vi "Update Non-SD Subpanel.vi"(7 "SubPanel Command":refnum<user-event>, 8 "error in (no error)":errorcluster, 9 "SubPanel Ref":refnum<vi>, 10 "SD Module in":refnum<class "SD Module.lvclass">, 11 "Node Ptr In":T1 format="%.0x") -> (0 "error out":errorcluster, 2 "SD Module out":refnum<class "SD Module.lvclass">, 3 "Node Ptr Out":T1 format="%.0x")   [LabVIEW 2017, in "Modules.lvlib" / "SD Module.lvclass"]
uses:
  SD Module.lvclass
  <vilib>/NI Veristand/Custom Device API/Custom Device Item Ref.ctl
  RSI Module/SubPanel Command.ctl
  <vilib>/Utility/miscctls.llb/LVRectTypeDef.ctl
  <vilib>/NI Veristand/Custom Device API/Custom Device API.lvlib
  RSI Module/RSI Module.lvclass
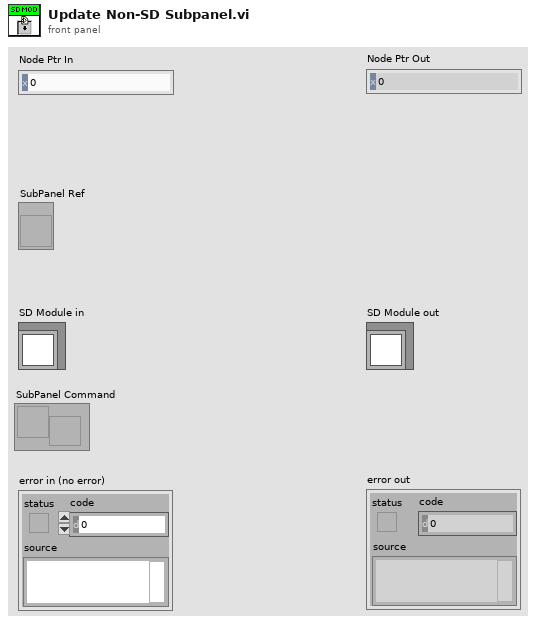
[diagram p1: front panel]
types:
  T1 = typedef "Custom Device API.lvlib/Custom Device Item Ref.ctl" = u64
  T2 = typedef "LVRectTypeDef.ctl" = cluster{"Left":i16, "Top":i16, "Right":i16, "Bottom":i16}
  T3 = typedef "LVBoundsTypeDef.ctl" = cluster{"Width":u32, "Height":u32}
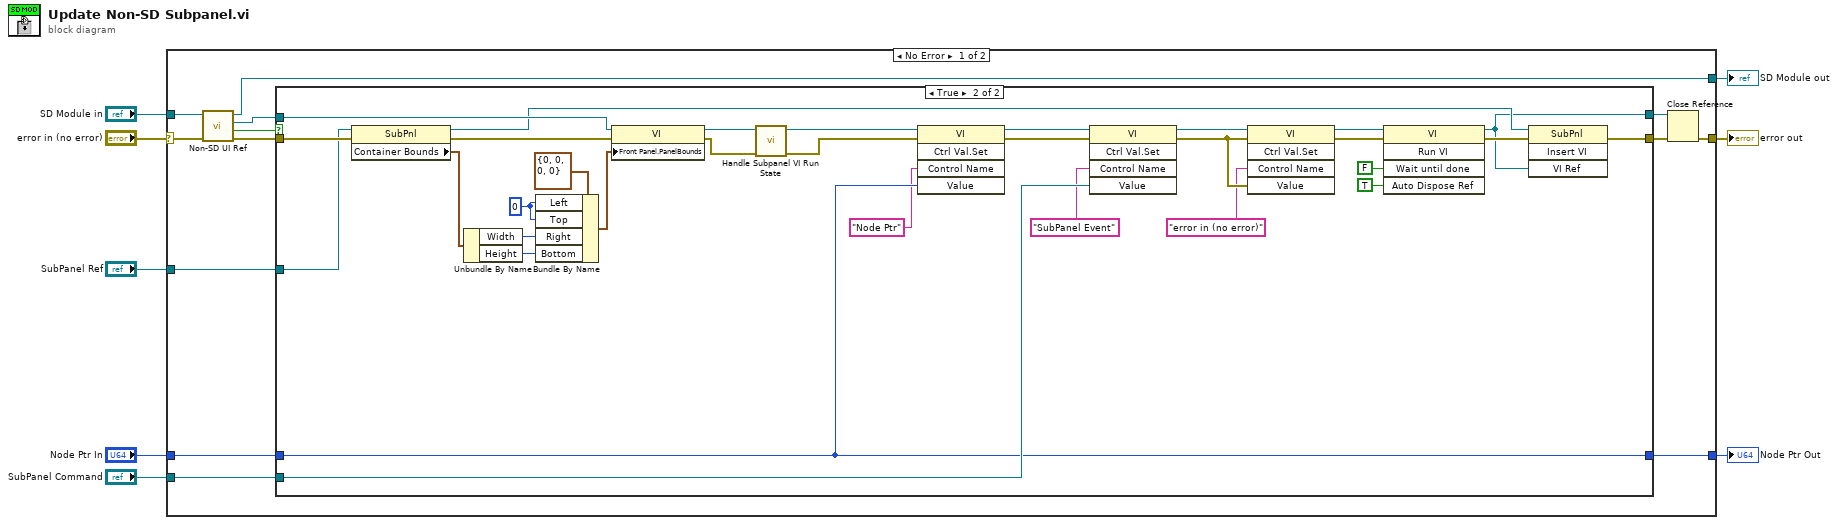
[diagram p0: block diagram]
diagram:
  n1 = case shown="No Error" "error in (no error)" {
    selector: "error in (no error)" -> [w11 w58]
    tunnel: "SubPanel Ref" -> [w21 _]
    tunnel: [w17 w58] -> w3
    tunnel: "Node Ptr In" -> [w16 w57]
    tunnel: "SubPanel Command" -> [w14 _]
    tunnel: "SD Module in" -> [w13 w56]
    tunnel: [w12 w56] -> w6
    tunnel: [w9 w57] -> w8
    frame No Error {
      n2 = call-dynamic "Non-SD UI Ref.vi"("error in (no error)"=w11, "SD Module in"=w13) -> ("error out"=w15:errorcluster, "Show SubPanel?"=w10:bool, "VI Refnum"=w20:refnum<vi>, "SD Module out"=w12:refnum<class "SD Module.lvclass">)  [unwired: 6 in]
      n3 = case shown="True" w10 {
        tunnel: w21 -> [_ w38]
        tunnel: w20 -> [w23 w50]
        tunnel: [w23 w32] -> w19
        tunnel: [w24 w33] -> w18
        tunnel: w16 -> [w22 w39]
        tunnel: w15 -> [w24 w42]
        tunnel: w14 -> [_ w40]
        tunnel: [w22 w39] -> w9
        frame False {
        }
        frame True {
          w53 = i16 0 ("Left")
          n4 = property class="SubPnl"(reference=w38, error in=w42) -> (reference out=w35:refnum<vi>, error out=w41:errorcluster, "Container Bounds"=w51:T3)
          n5 = Unbundle By Name(w51) -> ("Width"=w54:u32, "Height"=w55:u32)
          n6 = Bundle By Name(cluster=T2 {"Left"=0, "Top"=0, "Right"=0, "Bottom"=0} ("Front Panel Window:Panel Bounds"), "Left"=w53, "Top"=w53, "Right"=w54, "Bottom"=w55) -> (w49:T2)
          n7 = property class="VI"(reference=w50, error in=w41, "Front Panel.PanelBounds"=w49) -> (reference out=w28:refnum<vi>, error out=w27:errorcluster)
          n8 = call "Handle Subpanel VI Run State.vi"("error in (no error)"=w27, "VI in"=w28) -> ("error out"=w25:errorcluster, "VI out"=w26:refnum<vi>)  [unwired: 8 in]
          n9 = invoke class="VI" method="Ctrl Val.Set"(reference=w26, error in=w25, "Control Name"="Node Ptr" ("Node Ptr"), "Value"=w39) -> (reference out=w48:refnum<vi>, error out=w47:errorcluster)  [unwired: 1 in, 3 out]
          n10 = invoke class="VI" method="Ctrl Val.Set"(reference=w48, error in=w47, "Control Name"="SubPanel Event" ("SubPanel Event"), "Value"=w40) -> (reference out=w37:refnum<vi>, error out=w36:errorcluster)  [unwired: 1 in, 3 out]
          n11 = invoke class="VI" method="Ctrl Val.Set"(reference=w37, error in=w36, "Control Name"="error in (no error)" ("error in (no error)"), "Value"=w36) -> (reference out=w46:refnum<vi>, error out=w45:errorcluster)  [unwired: 1 in, 3 out]
          n12 = invoke class="VI" method="Run VI"(reference=w46, error in=w45, "Wait until done"=FALSE ("Wait Until Done"), "Auto Dispose Ref"=TRUE ("Auto Dispose Reference")) -> (reference out=w32:refnum<vi>, error out=w34:errorcluster)  [unwired: 1 in, 3 out]
          n13 = invoke class="SubPnl" method="Insert VI"(reference=w35, error in=w34, "VI Ref"=w32) -> (error out=w33:errorcluster)  [unwired: 1 in, 3 out]
        }
      }
      n14 = Close Reference(reference=w19, error in (no error)=w18) -> (error out=w17:errorcluster)
    }
    frame Error {
    }
  }
  "error out" <- w3
  "Node Ptr Out" <- w8
  "SD Module out" <- w6
